vi "set_channel_offsets.vi"(8 "error in (no error)":errorcluster, 10 "pixel values cluster":T1, 11 "FPGA_AK101022Resonance in":refnum<class "FPGAWrapperAK101022Resonance.lvclass">) -> (0 "error out":errorcluster, 3 "FPGA_AK101022Resonance out":refnum<class "FPGAWrapperAK101022Resonance.lvclass">)   [LabVIEW 2010]
uses:
  FPGAWrapperAK101022Resonance.lvclass
  common_typedefs/channels_cluster.ctl
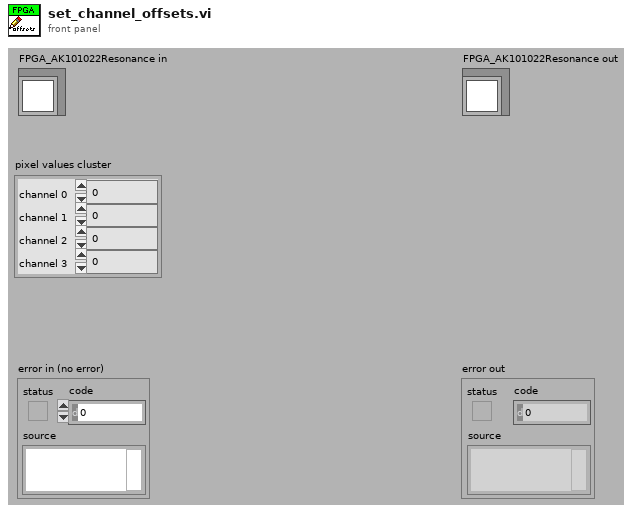
[diagram p1: front panel]
types:
  T1 = typedef "channels_cluster.ctl" = cluster{"channel 0":u32, "channel 1":u32, "channel 2":u32, "channel 3":u32}
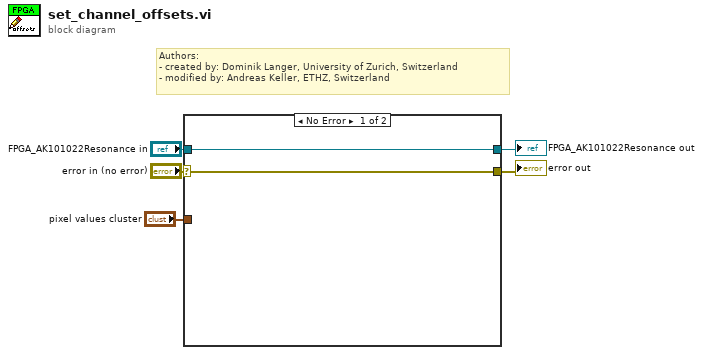
[diagram p0: block diagram]
diagram:
  # "Authors: \n- created by: Dominik Langer, University of Zurich, Switzerland\n- modified by: Andreas Keller, ETHZ, Switzerland"
  n1 = case shown="No Error" "error in (no error)" {
    selector: "error in (no error)" -> [w7 w8]
    tunnel: "FPGA_AK101022Resonance in" -> [w6 w9]
    tunnel: [w7 w8] -> w3
    tunnel: [w6 w9] -> w2
    tunnel: "pixel values cluster" -> [_ _]
    frame No Error {
    }
    frame Error {
    }
  }
  "error out" <- w3
  "FPGA_AK101022Resonance out" <- w2
